vi "init RxTx.vi"(8 "error in (no error)":errorcluster, 11 "Header content in":refnum<class "Header content.lvclass">) -> (0 "error out":errorcluster, 3 "Header content out":refnum<class "Header content.lvclass">)   [LabVIEW 2018, in "Header content.lvclass"]
uses:
  Header content.lvclass
  RxTx/RxTx.lvclass
  Header content.lvclass/Header content.ctl
panel:
  in  "RxTx in":refnum<class "RxTx.lvclass">
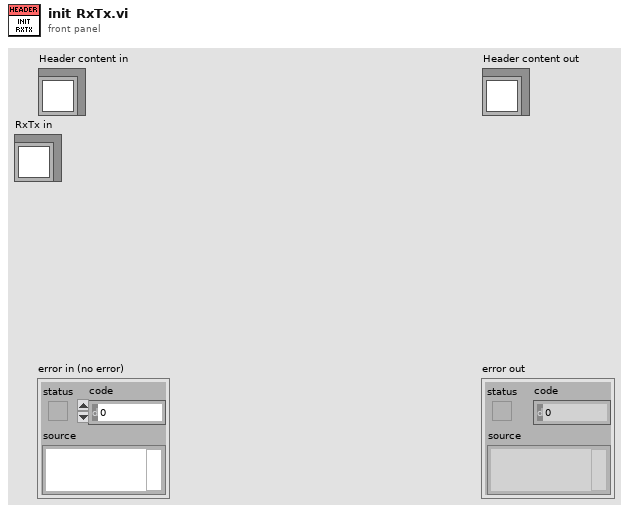
[diagram p1: front panel]
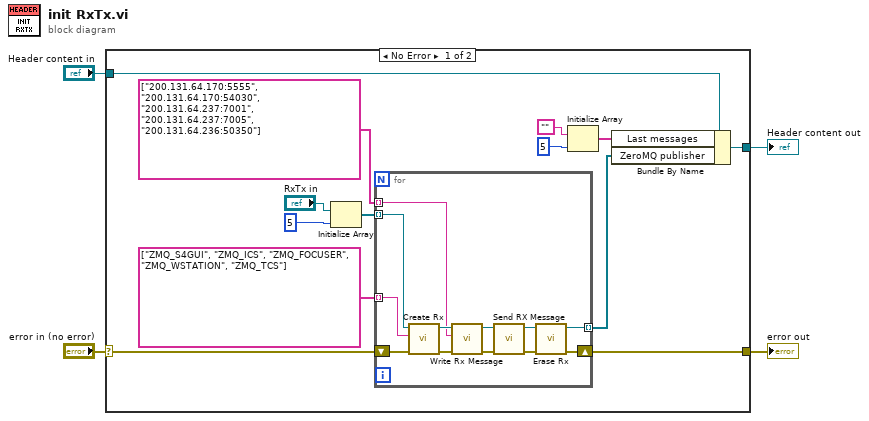
[diagram p0: block diagram]
diagram:
  n1 = case shown="No Error" "error in (no error)" {
    selector: "error in (no error)" -> [w17 w31]
    tunnel: [w16 w31] -> w3
    tunnel: [w13 w30] -> w1
    tunnel: "Header content in" -> [w15 w30]
    frame No Error {
      n2 = Initialize Array("RxTx in", 5 ("dimension size")) -> (w8:refnum<class "RxTx.lvclass">[])
      n3 = for {
        shift-right: [w21] -> w16
        shift-left: w17 -> [w29]
        tunnel: [w20] -> w14 mode=indexing
        tunnel: string[] ["ZMQ_S4GUI", "ZMQ_ICS", "ZMQ_FOCUSER", "ZMQ_WSTATION", "ZMQ_TCS"] -> [w28] mode=indexing
        tunnel: string[] ["200.131.64.170:5555", "200.131.64.170:54030", "200.131.64.237:7001", "200.131.64.237:7005", "200.131.64.236:50350"] -> [w23] mode=indexing
        tunnel: w8 -> [w18] mode=indexing
        n4 = call "Create Rx.vi"("error in (no error)"=w29, "Reader Name"=w28, "RxTx in"=w18) -> ("error out"=w27:errorcluster, "RxTx out"=w24:refnum<class "RxTx.lvclass">)  [unwired: 7 in]
        n5 = call "Write Rx Message.vi"("error in (no error)"=w27, "Rx Message"=w23, "RxTx in"=w24) -> ("error out"=w26:errorcluster, "RxTx out"=w25:refnum<class "RxTx.lvclass">)  [unwired: 7 in]
        n6 = call "Send RX Message.vi"("error in (no error)"=w26, "RxTx in"=w25) -> ("error out"=w22:errorcluster, "RxTx out"=w19:refnum<class "RxTx.lvclass">)  [unwired: 8 in]
        n7 = call "Erase Rx.vi"("error in (no error)"=w22, "RxTx in"=w19) -> ("error out"=w21:errorcluster, "RxTx out"=w20:refnum<class "RxTx.lvclass">)  [unwired: 8 in]
      }
      n8 = Initialize Array("", 5 ("dimension size")) -> (w5:string[])
      n9 = Bundle By Name(cluster=w15, "Last messages"=w5, "ZeroMQ publisher"=w14) -> (w13:refnum<class "Header content.lvclass">)
    }
    frame Error {
    }
  }
  "error out" <- w3
  "Header content out" <- w1
